vi "Flatten UIP Value.vi"(11 "Template UIP In":refnum<class "PositionUIP.lvclass">) -> (0 "Error Out":errorcluster, 2 "String Value":string, 3 "Template UIP Out":refnum<class "PositionUIP.lvclass">)   [LabVIEW 2020, in "UIM.lvlib" / "PositionUIP.lvclass"]
uses:
  PositionUIP.lvclass
  PositionUIP.lvclass/PositionUIP.ctl
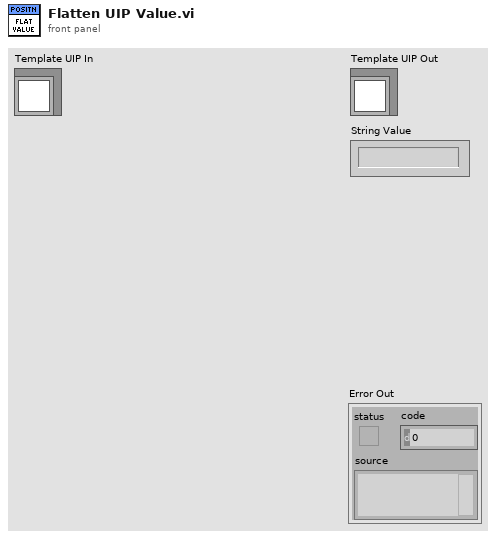
[diagram p1: front panel]
types:
  T1 = typedef "LVPositionTypeDef.ctl" = cluster{"Left":i32, "Top":i32}
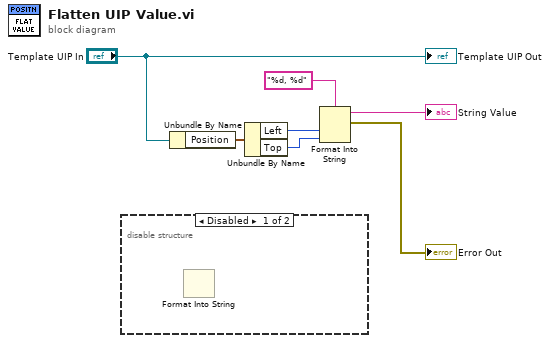
[diagram p0: block diagram]
diagram:
  n1 = disable-structure shown="Disabled" {
    frame Disabled {
      n2 = Format Into String "Format Into String"() -> ()  [unwired: 4 in, 2 out]
    }
    frame Enabled {
    }
  }
  n3 = Unbundle By Name("Template UIP In") -> ("Position"=w6:T1)
  n4 = Unbundle By Name(w6) -> ("Left"=w5:i32, "Top"=w4:i32)
  n5 = Format Into String(format string="%d, %d", w5, w4) -> (resulting string=→"String Value":string, error out=→"Error Out":errorcluster)  [unwired: 2 in]
  "Template UIP Out" <- "Template UIP In"
